vi "Init UserPrefs.vi"(8 "error in (no error)":errorcluster, 11 "BluelinesRedlines in":refnum<class "BluelinesRedlines.lvclass">) -> (0 "error out":errorcluster, 3 "BluelinesRedlines out":refnum<class "BluelinesRedlines.lvclass">)   [LabVIEW 2020, in "VolatusGUIElements.lvlib" / "BluelinesRedlines.lvclass"]
uses:
  BluelinesRedlines.lvclass
  BluelinesRedlines.lvclass/BluelinesRedlines.ctl
  Volatus/VolatusAPI/VolatusAPI.lvclass/VolatusAPI.ctl
  lv-userprefs/User Prefs/PrefsDB/PrefsDB.lvclass
  Volatus/VolatusAPI/VolatusAPI.lvclass
  lv-userprefs/User Prefs/Pref Group/Pref Group.lvclass
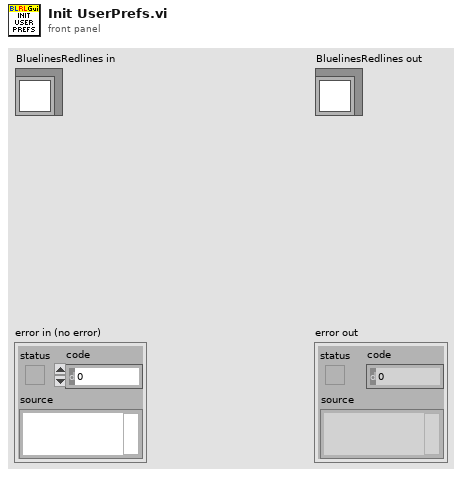
[diagram p1: front panel]
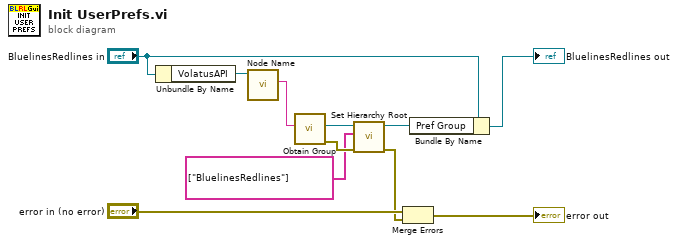
[diagram p0: block diagram]
diagram:
  n1 = Unbundle By Name("BluelinesRedlines in") -> ("VolatusAPI"=w9:refnum<class "VolatusAPI.lvclass">)
  n2 = call "Node Name.vi"("VolatusAPI in"=w9) -> ("Node Name"=w8:string)  [unwired: 8 in, 2 out]
  n3 = call "Obtain Group.vi"("Group"=w8) -> ("error out"=w6:errorcluster, "Pref Group"=w7:refnum<class "Pref Group.lvclass">)  [unwired: 8 in, 1 out]
  n4 = call "Set Hierarchy Root.vi"("error in (no error)"=w6, "Hierarchy Root"=string[] ["BluelinesRedlines"], "Pref Group in"=w7) -> ("error out"=w1:errorcluster, "Pref Group out"=w3:refnum<class "Pref Group.lvclass">)  [unwired: 7 in]
  n5 = Merge Errors("error in (no error)", w1) -> (→"error out":errorcluster)
  n6 = Bundle By Name(cluster="BluelinesRedlines in", "Pref Group"=w3) -> (→"BluelinesRedlines out":refnum<class "BluelinesRedlines.lvclass">)
